vi "Change Label.vi"() -> ()   [LabVIEW 2017]
uses:
  <vilib>/Utility/file.llb/Read Delimited Spreadsheet (string).vi
panel:
  out "Array 2":string[](array[string])
  out "Array":string[](array[string])
  out "first row":string[](array[string])
  in  "path":path
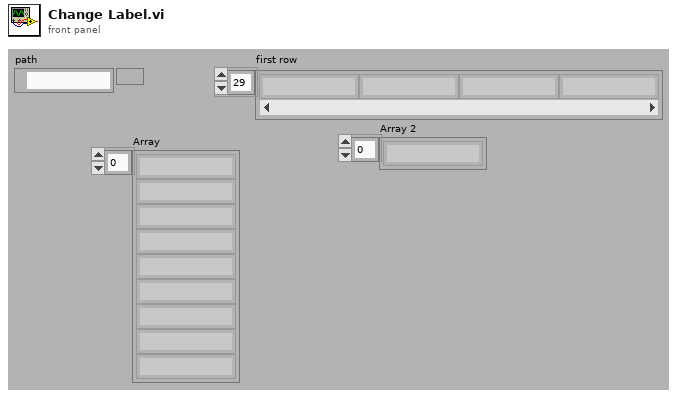
[diagram p1: front panel]
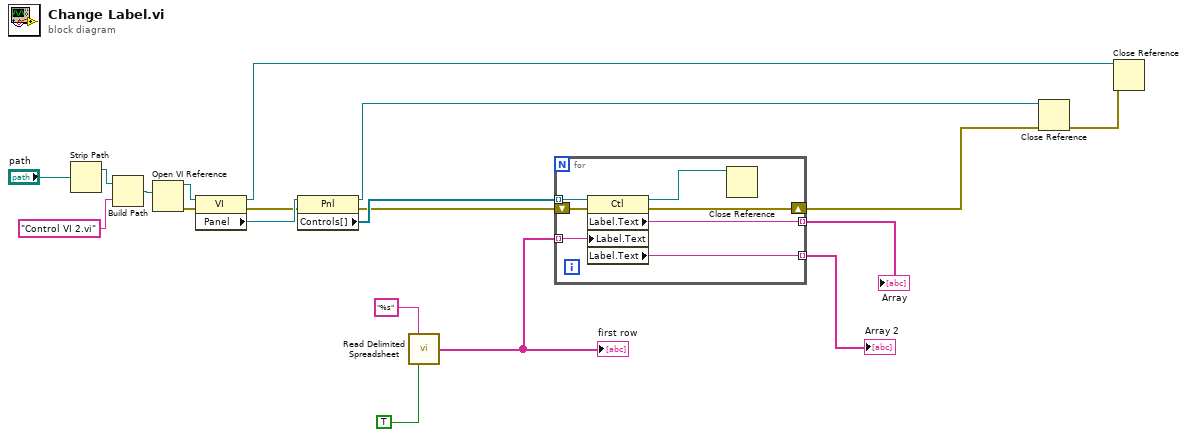
[diagram p0: block diagram]
diagram:
  n1 = Strip Path(path="path") -> (stripped path=w14:path)  [unwired: 1 out]
  n2 = Build Path(base path=w14, name or relative path="Control VI 2.vi") -> (appended path=w12:path)
  n3 = Open VI Reference(vi path=w12) -> (vi reference=w19:refnum<vi>, error out=w18:errorcluster)  [unwired: 5 in]
  n4 = property class="VI"(reference=w19, error in=w18) -> (reference out=w16:refnum<vi>, error out=w5:errorcluster, "Panel"=w17:refnum<vi>)
  n5 = property class="Pnl"(reference=w17, error in=w5) -> (reference out=w15:refnum<vi>, error out=w6:errorcluster, "Controls[]"=w10:refnum<vi>[])
  n6 = call-poly <vilib>:"Read Delimited Spreadsheet.vi"("format (%s)"="%s" ("format (%.3f)"), "transpose? (F)"=TRUE) -> ("first row"=w7:string[])  [unwired: 8 in, 5 out]
  "first row" <- w7
  n7 = for {
    tunnel: w7 -> [w23] mode=indexing
    shift-right: [w25] -> w2
    shift-left: w6 -> [w26]
    tunnel: w10 -> [w24] mode=indexing
    tunnel: [w22] -> w3 mode=indexing
    tunnel: [w20] -> w1 mode=indexing
    n8 = property class="Ctl"(reference=w24, error in=w26, "Label.Text"=w23) -> (reference out=w21:refnum<vi>, error out=w25:errorcluster, "Label.Text"=w22:string, "Label.Text"=w20:string)
    n9 = Close Reference(reference=w21) -> ()  [unwired: 1 in, 1 out]
  }
  "Array" <- w3
  "Array 2" <- w1
  n10 = Close Reference(reference=w15, error in (no error)=w2) -> (error out=w4:errorcluster)
  n11 = Close Reference(reference=w16, error in (no error)=w4) -> ()  [unwired: 1 out]
